vi "Cleanup Channels.vi"(8 "error in (no error)":errorcluster, 11 "Output Sequencer In":refnum<class "Output Sequencer.lvclass">) -> (0 "error out":errorcluster, 1 "Num of Digital Channels":i32, 2 "Num of Analog Channels":i32, 3 "Output Sequencer out":refnum<class "Output Sequencer.lvclass">)   [LabVIEW 2024, in "Output Sequencer.lvlib" / "Output Sequencer.lvclass"]
uses:
  Output Sequencer.lvclass
  C:/Program Files/National Instruments/LabVIEW 2024/vi.lib/FlexLogger/SDK/PluginSDK.lvlibp/PEFClasses/SDK/Plugin/Plugin.lvclass
  <vilib>/FlexLogger/SDK/PluginSDK.lvlibp/PEFClasses/SDK/Channel/Data Type_v2.ctl
  Output Sequencer.lvclass/Output Sequencer.ctl
  Globals/Global Strings.vi
  <vilib>/FlexLogger/SDK/PluginSDK.lvlibp/PEFClasses/SDK/Plugin/Read Channels.vi
  <vilib>/FlexLogger/SDK/PluginSDK.lvlibp/PEFClasses/SDK/Channel/Channel.lvclass
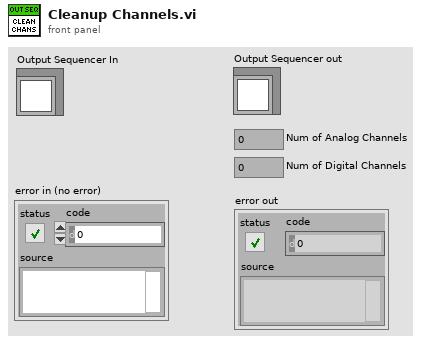
[diagram p1: front panel]
types:
  T1 = typedef "PluginSDK.lvlibp/Channel.lvclass/Data Type_v2.ctl" = u16
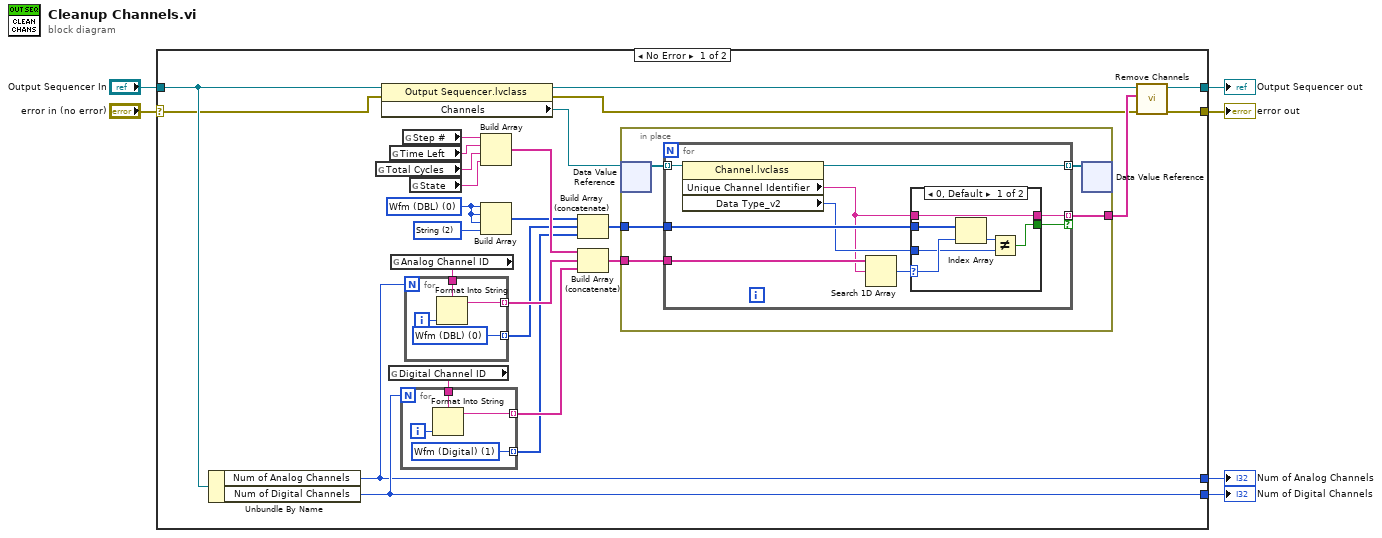
[diagram p0: block diagram]
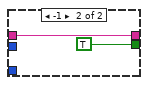
[diagram p2: hidden frame]
diagram:
  n1 = case shown="No Error" "error in (no error)" {
    selector: "error in (no error)" -> [w7 w63]
    tunnel: [w32 w63] -> w6
    tunnel: [w31 w64] -> w5
    tunnel: [w30 _] -> w4
    tunnel: "Output Sequencer In" -> [w29 w64]
    tunnel: [w28 _] -> w2
    frame No Error {
      w13 = T1 2 items=["Wfm (DBL)", "Wfm (Digital)", "String"] ("Data Type_v2")
      w8 = T1 0 items=["Wfm (DBL)", "Wfm (Digital)", "String"] ("Data Type_v2")
      n2 = Unbundle By Name(w29) -> ("Num of Analog Channels"=w28:i32, "Num of Digital Channels"=w30:i32)
      n3 = global read "Global Strings.vi" "Total Cycles"() -> (w20:string)
      n4 = property class="Output Sequencer.lvclass"(reference=w29, error in=w7) -> (reference out=w12:refnum<class "Output Sequencer.lvclass">, error out=w9:errorcluster, "Channels"=w11:refnum<data-value>)
      n5 = global read "Global Strings.vi" "Digital Channel ID"() -> (w24:string)
      n6 = global read "Global Strings.vi" "Time Left"() -> (w21:string)
      n7 = global read "Global Strings.vi" "Analog Channel ID"() -> (w25:string)
      n8 = for {
        N: w30 -> [_]
        tunnel: w24 -> [w61]
        tunnel: [w60] -> w18 mode=indexing
        tunnel: [w59] -> w15 mode=indexing
        i -> [w62]
        w59 = T1 1 items=["Wfm (DBL)", "Wfm (Digital)", "String"] ("Data Type_v2")
        n9 = Format Into String(format string=w61, w62) -> (resulting string=w60:string)  [unwired: 2 in, 1 out]
      }
      n10 = global read "Global Strings.vi" "Step #"() -> (w22:string)
      n11 = for {
        N: w28 -> [_]
        tunnel: w25 -> [w35]
        tunnel: [w34] -> w23 mode=indexing
        tunnel: [w33] -> w17 mode=indexing
        i -> [w36]
        w33 = T1 0 items=["Wfm (DBL)", "Wfm (Digital)", "String"] ("Data Type_v2")
        n12 = Format Into String(format string=w35, w36) -> (resulting string=w34:string)  [unwired: 2 in, 1 out]
      }
      n13 = global read "Global Strings.vi" "State"() -> (w14:string)
      n14 = Build Array(w22, w21, w20, w14) -> (w19:string[])
      n15 = Build Array(w8, w8, w8, w13) -> (w16:T1[])
      n16 = Build Array (concatenate)(w16, w17, w15) -> (w26:T1[])
      n17 = Build Array (concatenate)(w19, w23, w18) -> (w27:string[])
      n18 = in-place {
        in-place-border: [w40] -> w10
        in-place-border: w27 -> [w39]
        in-place-border: w26 -> [w38]
        n19 = in-place-dvr #1(w11) -> (w41:refnum<class "Channel.lvclass">[])  [unwired: 1 out]
        n20 = for {
          tunnel: w41 -> [w50] mode=indexing
          tunnel: [w43] -> w40 mode=indexing if=w47
          tunnel: w39 -> [w49]
          tunnel: w38 -> [w46]
          tunnel: [w42] -> w37 mode=indexing
          n21 = property class="Channel.lvclass"(reference=w50) -> (reference out=w42:refnum<class "Channel.lvclass">, "Unique Channel Identifier"=w44:string, "Data Type_v2"=w45:T1)  [unwired: 1 in, 1 out]
          n22 = Search 1D Array(1D array=w49, element=w44) -> (index of element=w48:i32)  [unwired: 1 in]
          n23 = case shown="0, Default" w48 {
            selector: w48 -> [w55 _]
            tunnel: [w52 TRUE] -> w47
            tunnel: w46 -> [w56 _]
            tunnel: w45 -> [w54 _]
            tunnel: w44 -> [w51 w57]
            tunnel: [w51 w57] -> w43
            frame 0, Default {
              n24 = Index Array(array=w56, index=w55) -> (element=w53:T1)
              n25 = Not Equal?(x=w53, y=w54) -> (x != y?=w52:bool)
            }
            frame -1 {
            }
          }
        }
        n26 = in-place-dvr #1(w37) -> ()  [unwired: 2 out]
      }
      n27 = call-dynamic "Remove Channels.vi"("error in (no error)"=w9, "Unique Channel Identifiers to Delete"=w10, "Plugin in"=w12) -> ("error out"=w32:errorcluster, "Plugin out"=w31:refnum<class "Output Sequencer.lvclass">)  [unwired: 7 in]
    }
    frame Error {
    }
  }
  "Num of Analog Channels" <- w2
  "Num of Digital Channels" <- w4
  "error out" <- w6
  "Output Sequencer out" <- w5
